vi "make_cursor_main.vi"(4 "Scale":T3, 6 "Track Eye":T4, 7 "Cursor Properties":T10={"Cursor Visible"=FALSE, "Cursor Enable"=FALSE, "Cursor Point"={"Point Color"=0, "Point Size"=0.0, "Point Visible"=FALSE}, "Cursor Position"={"Position X"=0.0, "Position Y"=0.0, "Position Z"=0.0, "Position Snap To"=enum."Fixed", "Polsition Pick Plot"=0, "Position Column"=0, "Position Row"=0}, "Cursor Line"={"Line Color"=0, "Line Width"=0.0, "Line Visible"=FALSE}, "Cursor Plane"={"Plane Opacity"=0.0, "Plane Color"=0, "Plane YZ"=FALSE, "Plane XZ"=FALSE, "Plane XY"=FALSE}, "Cursor Name"="", "Cursor Text"={"Cursor Name"="Cursor0", "Font Size"=7, "Show Position"=TRUE, "Show Name"=TRUE, "Text Color"=0, "Back Color"=16754450, "Opacity"=0.5}}, 8 "Actual Range Min/Max":T1, 11 "Scene Cursor Object In":refnum<vi>) -> (3 "Scene Cursor Object Out":refnum<vi>)   [LabVIEW 2020, in "3DPC_SurfacePlot.xctl"]
uses:
  <vilib>/Native 3D Graph/xcontrol/3DPC_SurfacePlot.xctl
  <vilib>/Native 3D Graph/typedefs/prop_cursor_point.ctl
  <vilib>/Native 3D Graph/typedefs/prop_cursor_position.ctl
  <vilib>/Native 3D Graph/typedefs/prop_cursor_line.ctl
  <vilib>/Native 3D Graph/typedefs/prop_cursor_plane.ctl
  <vilib>/Native 3D Graph/typedefs/prop_cursor_text.ctl
  <vilib>/Native 3D Graph/typedefs/track_eye.ctl
  <vilib>/Native 3D Graph/typedefs/vector.ctl
  <vilib>/Native 3D Graph/typedefs/range_cluster.ctl
  <vilib>/Native 3D Graph/typedefs/min_max.ctl
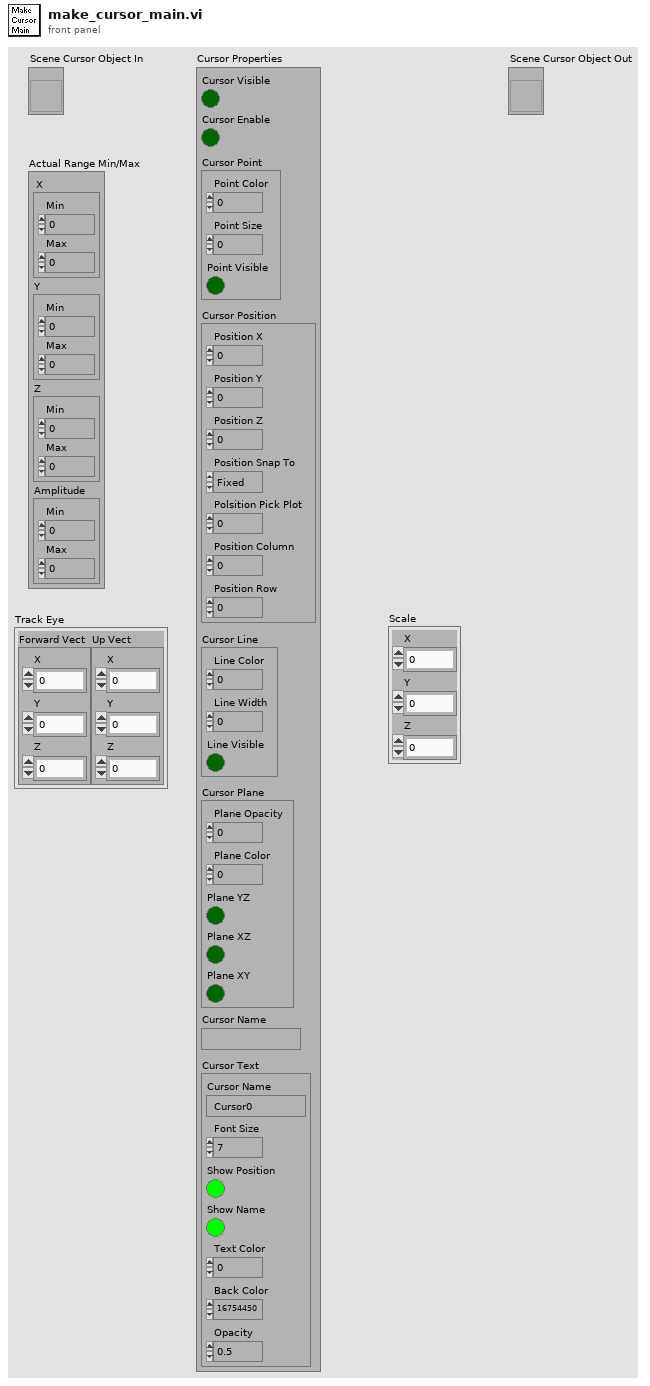
[diagram p1: front panel]
types:
  T1 = typedef "3DPC_SurfacePlot.xctl/range_cluster.ctl" = cluster{"X":T2, "Y":T2, "Z":T2, "Amplitude":T2}
  T2 = typedef "3DPC_SurfacePlot.xctl/min_max.ctl" = cluster{"Min":sgl, "Max":sgl}
  T3 = typedef "3DPC_SurfacePlot.xctl/vector.ctl" = cluster{"X":sgl, "Y":sgl, "Z":sgl}
  T4 = typedef "3DPC_SurfacePlot.xctl/track_eye.ctl" = cluster{"Forward Vect":T3, "Up Vect":T3}
  T5 = typedef "3DPC_SurfacePlot.xctl/prop_cursor_point.ctl" = cluster{"Point Color":u32, "Point Size":dbl, "Point Visible":bool}
  T6 = typedef "3DPC_SurfacePlot.xctl/prop_cursor_position.ctl" = cluster{"Position X":dbl, "Position Y":dbl, "Position Z":dbl, "Position Snap To":enum16{"Fixed", "Nearest Plot", "Snap to Plot"}, "Polsition Pick Plot":u16, "Position Column":i32, "Position Row":i32}
  T7 = typedef "3DPC_SurfacePlot.xctl/prop_cursor_line.ctl" = cluster{"Line Color":u32, "Line Width":dbl, "Line Visible":bool}
  T8 = typedef "3DPC_SurfacePlot.xctl/prop_cursor_plane.ctl" = cluster{"Plane Opacity":dbl, "Plane Color":u32, "Plane YZ":bool, "Plane XZ":bool, "Plane XY":bool}
  T9 = typedef "3DPC_SurfacePlot.xctl/prop_cursor_text.ctl" = cluster{"Cursor Name":string, "Font Size":i32, "Show Position":bool, "Show Name":bool, "Text Color":u32, "Back Color":u32, "Opacity":dbl}
  T10 = cluster{"Cursor Visible":bool, "Cursor Enable":bool, "Cursor Point":T5, "Cursor Position":T6, "Cursor Line":T7, "Cursor Plane":T8, "Cursor Name":string, "Cursor Text":T9}
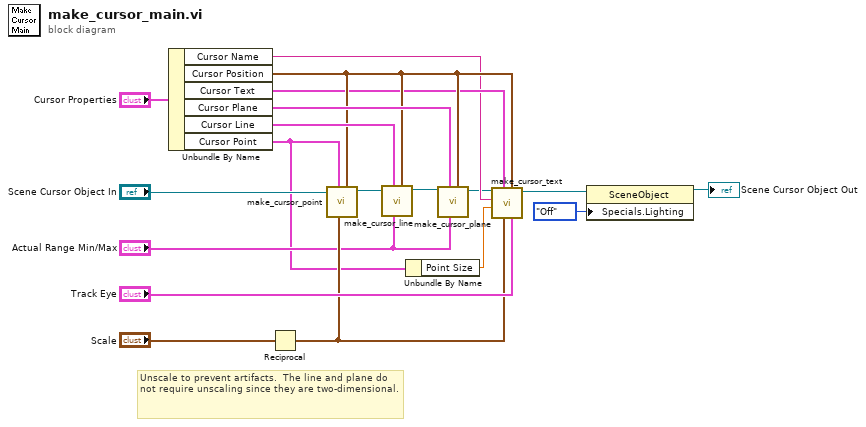
[diagram p0: block diagram]
diagram:
  # "Unscale to prevent artifacts.  The line and plane do not require unscaling since they are two-dimensional."
  n1 = Unbundle By Name("Cursor Properties") -> ("Cursor Name"=w9:string, "Cursor Position"=w12:T6, "Cursor Text"=w10:T9, "Cursor Plane"=w15:T8, "Cursor Line"=w16:T7, "Cursor Point"=w2:T5)
  n2 = Reciprocal(x="Scale") -> (1/x=w7:T3)
  n3 = call <vilib>:"make_cursor_point.vi"("Cursor Position"=w12, "Scale"=w7, "Cursor Point"=w2, "Scene Cursor Object In"="Scene Cursor Object In") -> ("Scene Cursor Object Out"=w5:refnum<vi>)  [unwired: 7 out]
  n4 = call <vilib>:"make_cursor_line.vi"("Cursor Position"=w12, "Actual Range Min/Max"="Actual Range Min/Max", "Cursor Line"=w16, "Scene Cursor Object In"=w5) -> ("Scene Cursor Object Out"=w4:refnum<vi>)  [unwired: 7 out]
  n5 = Unbundle By Name(w2) -> ("Point Size"=w1:dbl)
  n6 = call <vilib>:"make_cursor_plane.vi"("Cursor Position"=w12, "Actual Range Min/Max"="Actual Range Min/Max", "Cursor Plane"=w15, "Scene Cursor Object In"=w4) -> ("Scene Cursor Object Out"=w3:refnum<vi>)  [unwired: 7 out]
  n7 = call <vilib>:"make_cursor_text.vi"("Track Eye"="Track Eye", "Cursor Position"=w12, "Scale"=w7, "Cursor Text"=w10, "Point Size"=w1, "Cursor Name"=w9, "Scene Cursor Object In"=w3) -> ("Scene Cursor Object Out"=w13:refnum<vi>)  [unwired: 1 in, 3 out]
  n8 = property class="SceneObject"(reference=w13, "Specials.Lighting"=enum16{"Inherit Value", "Off", "On"}."Off" ("Specials:Lighting")) -> (reference out=→"Scene Cursor Object Out":refnum<vi>)  [unwired: 1 in, 1 out]
